vi "From JSON String.vi"(8 "error in (no error)":errorcluster, 10 "String":string, 11 "IConfigure in":refnum<class "IConfigure.lvclass">) -> (0 "error out":errorcluster, 3 "IConfigure out":refnum<class "IConfigure.lvclass">)   [LabVIEW 2023, in "HAL Interfaces.lvlib" / "IConfigure.lvclass"]
uses:
  IConfigure.lvclass
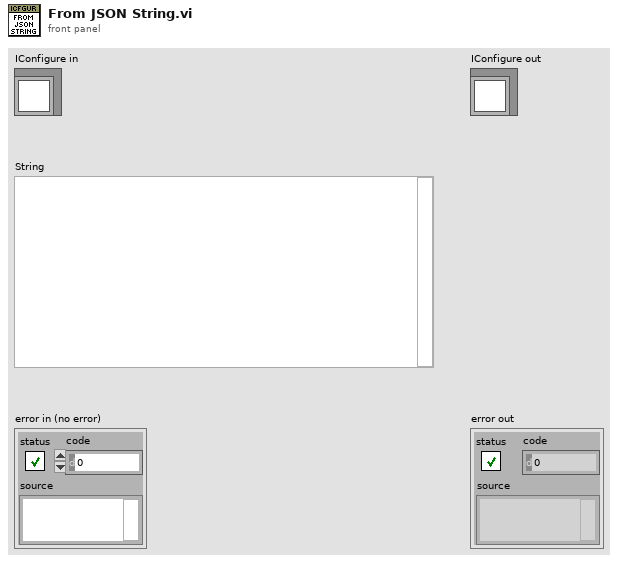
[diagram p1: front panel]
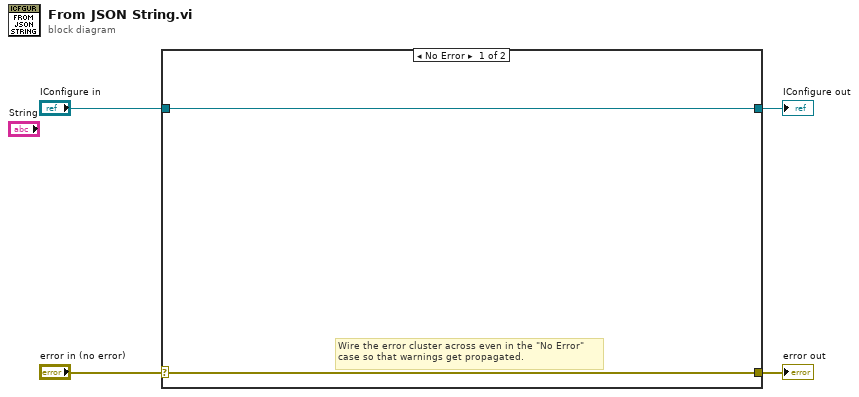
[diagram p0: block diagram]
diagram:
  n1 = case shown="No Error" "error in (no error)" {
    selector: "error in (no error)" -> [w5 w8]
    tunnel: [w5 w8] -> w3
    tunnel: [w6 w7] -> w1
    tunnel: "IConfigure in" -> [w6 w7]
    frame No Error {
      # "Wire the error cluster across even in the \"No Error\"\ncase so that warnings get propagated."
    }
    frame Error {
    }
  }
  "error out" <- w3
  "IConfigure out" <- w1
